vi "TCPGetMulliganList.vi"(1 "error in (no error)":errorcluster, 4 "connection ID":refnum<k5>) -> ()   [LabVIEW 2013]
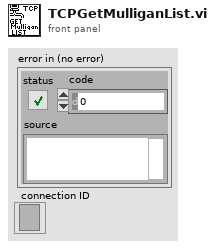
[diagram p1: front panel]
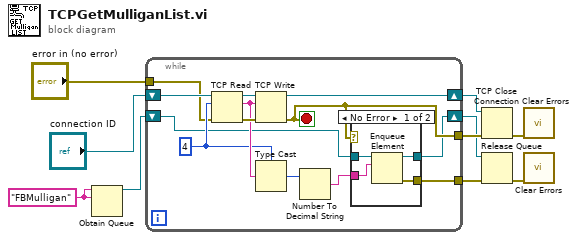
[diagram p0: block diagram]
diagram:
  w5 = "FBMulligan" ("name (unnamed)")
  n1 = Obtain Queue(name (unnamed)=w5, element data type=w5) -> (queue out=w4:refnum<queue>)  [unwired: 3 in, 2 out]
  n2 = while {
    tunnel: [w15] -> w10
    shift-right: [w21] -> w9
    shift-left: "connection ID" -> [w18]
    tunnel: "error in (no error)" -> [w16]
    shift-right: [w12] -> w3
    shift-left: w4 -> [w14]
    tunnel: [w11] -> w2
    stop <- w15 stop-if-true
    w17 = 4
    n3 = TCP Read(connection ID=w18, bytes to read=w17, error in (no error)=w16) -> (connection ID out=w22:refnum<k5>, data out=w20:string, error out=w23:errorcluster)  [unwired: 2 in]
    n4 = TCP Write(connection ID=w22, data in=w20, error in (no error)=w23) -> (connection ID out=w21:refnum<k5>, error out=w15:errorcluster)  [unwired: 1 in, 1 out]
    n5 = Type Cast(type=w17, x=w20) -> (*(type *) &x=w19:i32)
    n6 = Number To Decimal String(number=w19) -> (decimal integer string=w13:string)  [unwired: 1 in]
    n7 = case shown="No Error" w15 {
      tunnel: w14 -> [w26 w28]
      tunnel: w13 -> [w27 _]
      tunnel: [w25 w28] -> w12
      tunnel: [w24 _] -> w11
      frame No Error {
        n8 = Enqueue Element(queue=w26, element=w27) -> (queue out=w25:refnum<queue>, error out=w24:errorcluster)  [unwired: 2 in, 1 out]
      }
      frame Error {
      }
    }
  }
  n9 = TCP Close Connection(connection ID=w9, error in (no error)=w10) -> (error out=w8:errorcluster)  [unwired: 1 in, 1 out]
  n10 = Release Queue(queue=w3, error in (no error)=w2) -> (error out=w1:errorcluster)  [unwired: 1 in, 2 out]
  n11 = call <vilib>:"Clear Errors.vi"("error in (no error)"=w8) -> ()  [unwired: 6 in, 1 out]
  n12 = call <vilib>:"Clear Errors.vi"("error in (no error)"=w1) -> ()  [unwired: 6 in, 1 out]
